vi "Page_Advanced_Initialize.vi"(6 "ctl references":T1, 8 "error in (no error)":errorcluster, 11 "AB_DLL in":refnum<class "AB_DLL.lvclass">) -> (0 "error out":errorcluster, 3 "AB_DLL out":refnum<class "AB_DLL.lvclass">)   [LabVIEW 2020, in "AB_DLL.lvclass"]
uses:
  <vilib>/AppBuilder/AB_Classes/DLL/AB_DLL.lvclass
  <resource>/Framework/Providers/Builds/AppBuilder/AB_UI_Page_Advanced_References.ctl
  <resource>/Framework/Providers/Common/provcom_StringGlobals.vi
  <vilib>/AppBuilder/AB_Classes/Application/AB_Application.lvclass
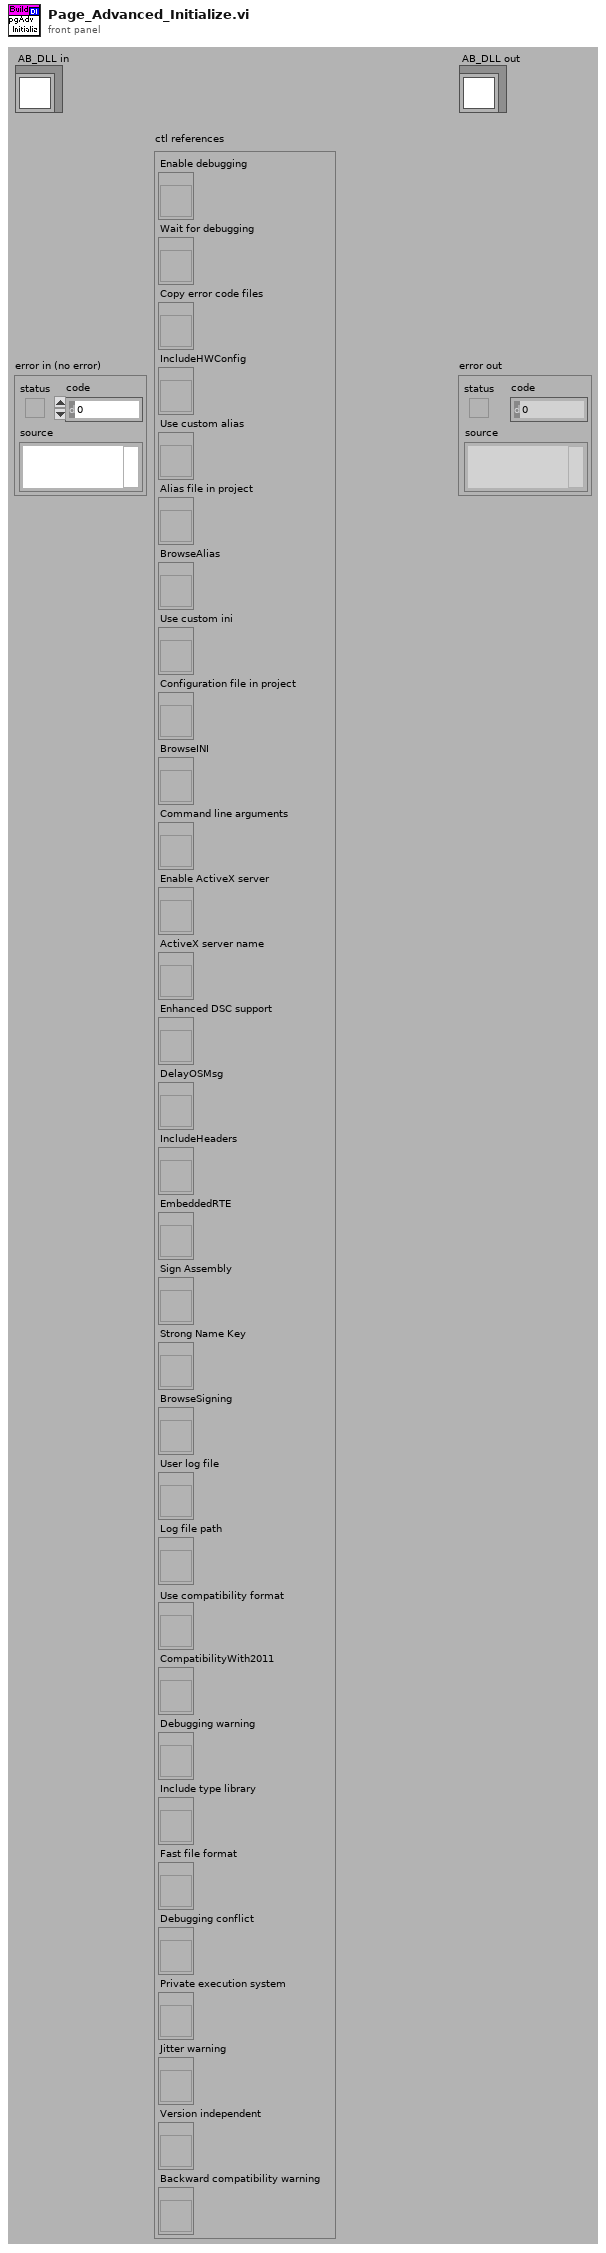
[diagram p1: front panel]
types:
  T1 = typedef "AB_UI_Page_Advanced_References.ctl" = cluster{"Enable debugging":refnum<vi>, "Wait for debugging":refnum<vi>, "Copy error code files":refnum<vi>, "IncludeHWConfig":refnum<vi>, "Use custom alias":refnum<vi>, "Alias file in project":refnum<vi>, "BrowseAlias":refnum<vi>, "Use custom ini":refnum<vi>, "Configuration file in project":refnum<vi>, "BrowseINI":refnum<vi>, "Command line arguments":refnum<vi>, "Enable ActiveX server":refnum<vi>, "ActiveX server name":refnum<vi>, "Enhanced DSC support":refnum<vi>, "DelayOSMsg":refnum<vi>, "IncludeHeaders":refnum<vi>, "EmbeddedRTE":refnum<vi>, "Sign Assembly":refnum<vi>, "Strong Name Key":refnum<vi>, "BrowseSigning":refnum<vi>, "User log file":refnum<vi>, "Log file path":refnum<vi>, "Use compatibility format":refnum<vi>, "CompatibilityWith2011":refnum<vi>, "Debugging warning":refnum<vi>, "Include type library":refnum<vi>, "Fast file format":refnum<vi>, "Debugging conflict":refnum<vi>, "Private execution system":refnum<vi>, "Jitter warning":refnum<vi>, "Version independent":refnum<vi>, "Backward compatibility warning":refnum<vi>}
  T2 = enum32{"invalid OS target", "Mac OS", "Windows 3.1", "Windows 95/NT", "Solaris 1", "Solaris 2", "HP-UX", "PowerMAX", "Linux", "Irix", "Rhapsody", "BeOS", "AIX", "OSF1", "VxWorks", "PharLap", "Carbon", "RTX", "Windows x64", "Linux x64", "Mac OS X x64"}
  T3 = typedef "LVRectTypeDef.ctl" = cluster{"Left":i16, "Top":i16, "Right":i16, "Bottom":i16}
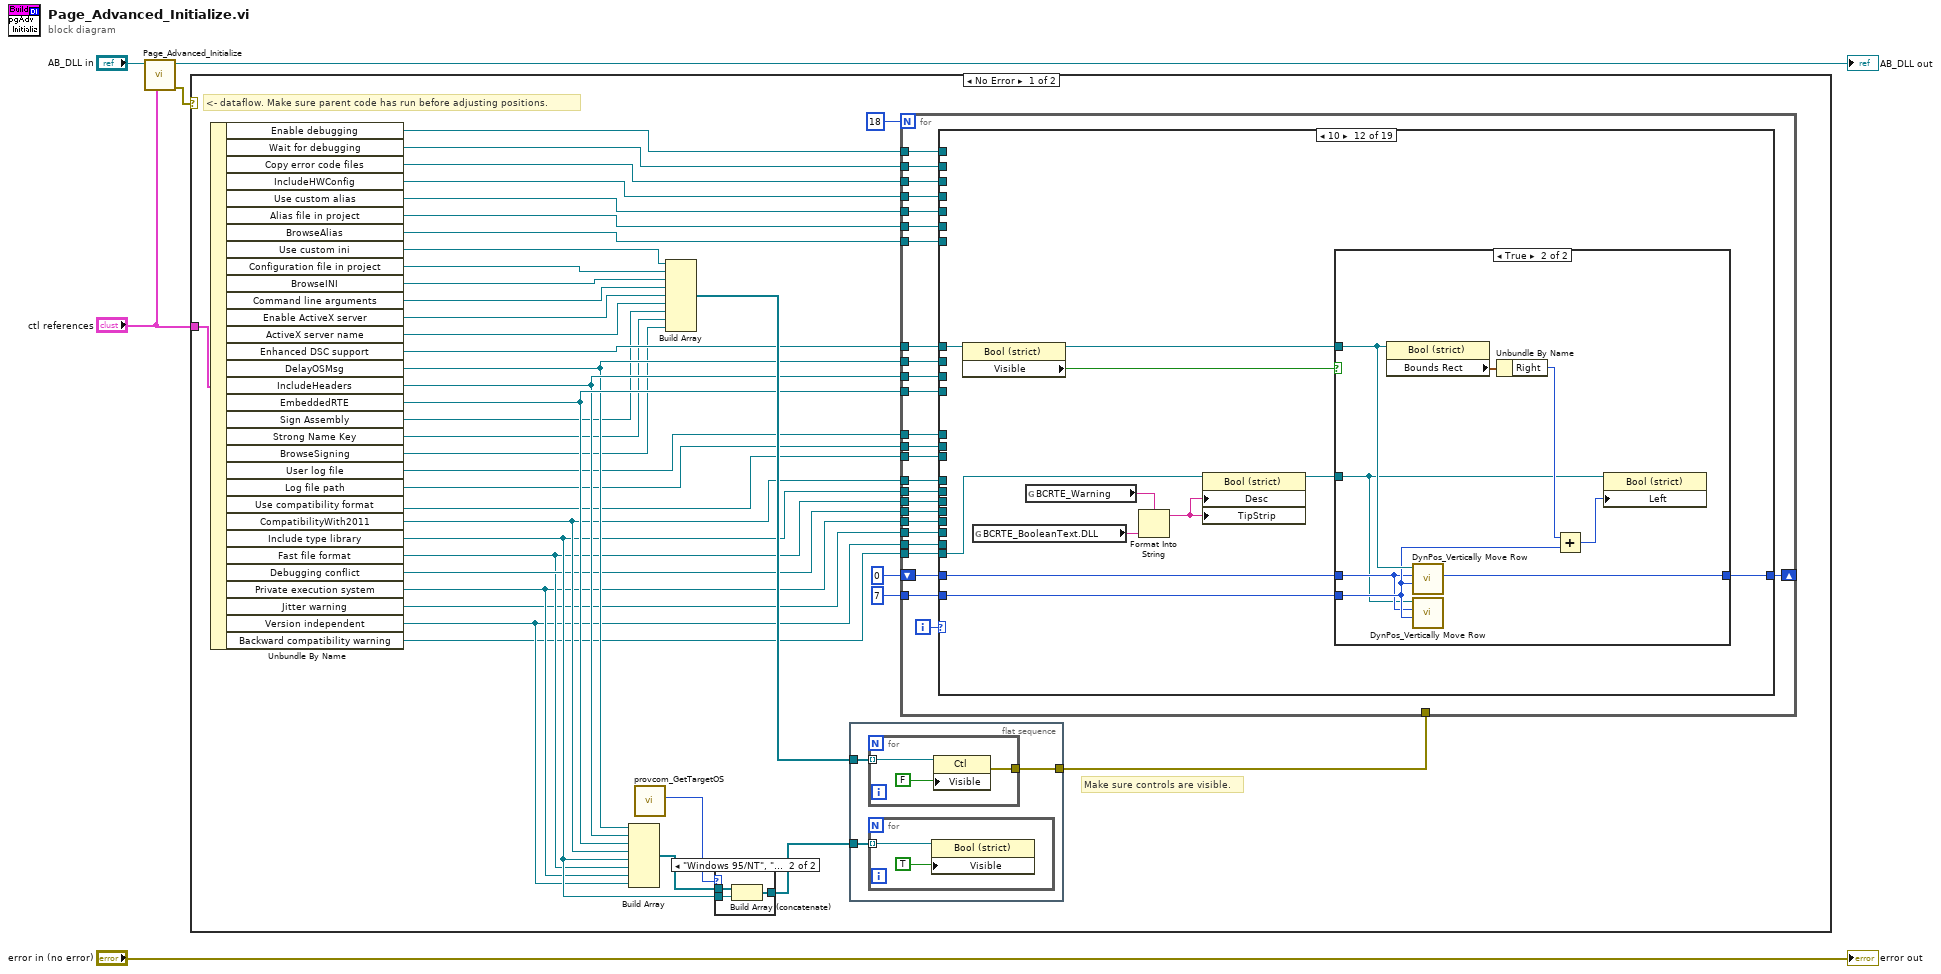
[diagram p0: block diagram]
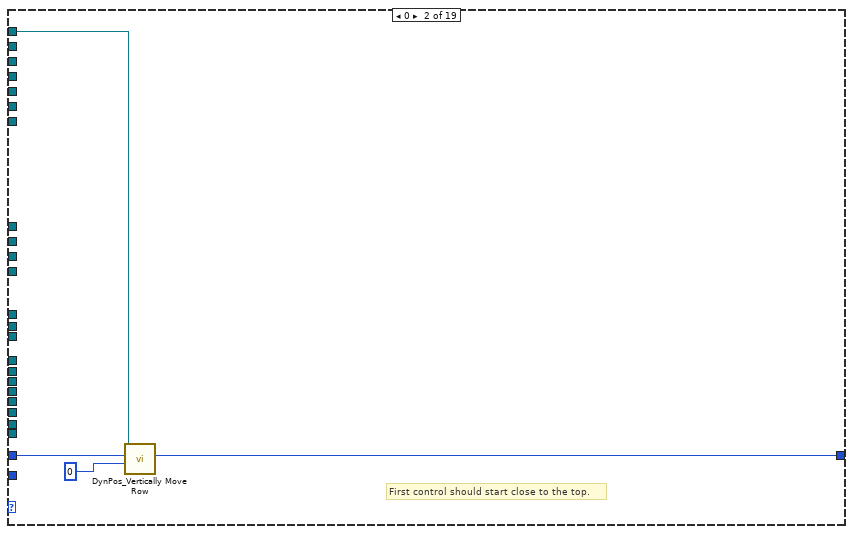
[diagram p4: hidden frame]
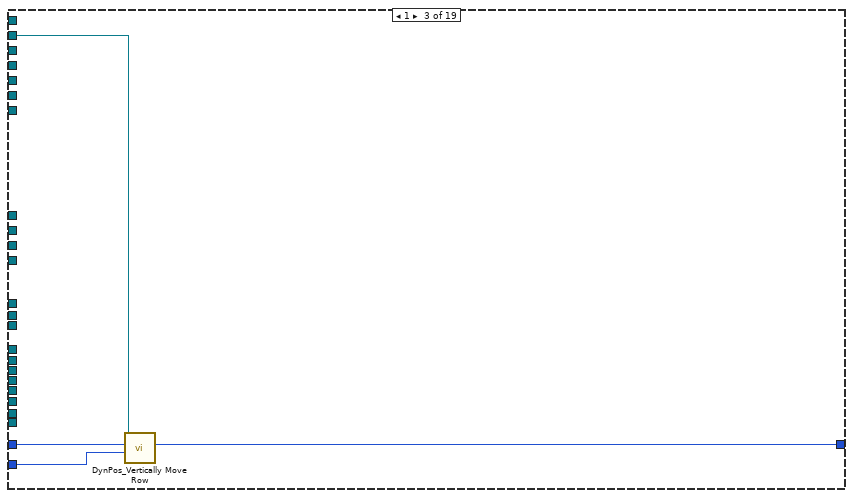
[diagram p5: hidden frame]
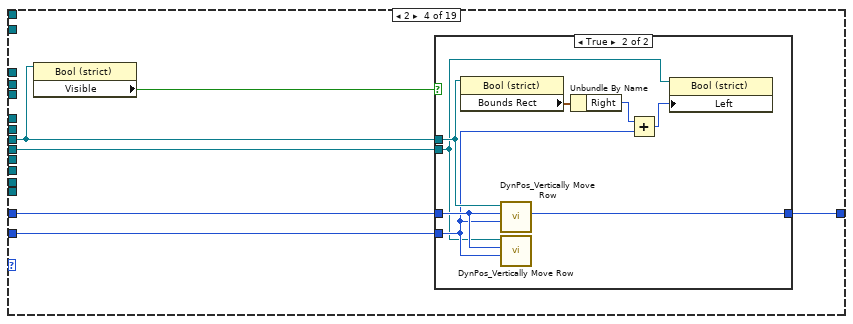
[diagram p6: hidden frame]
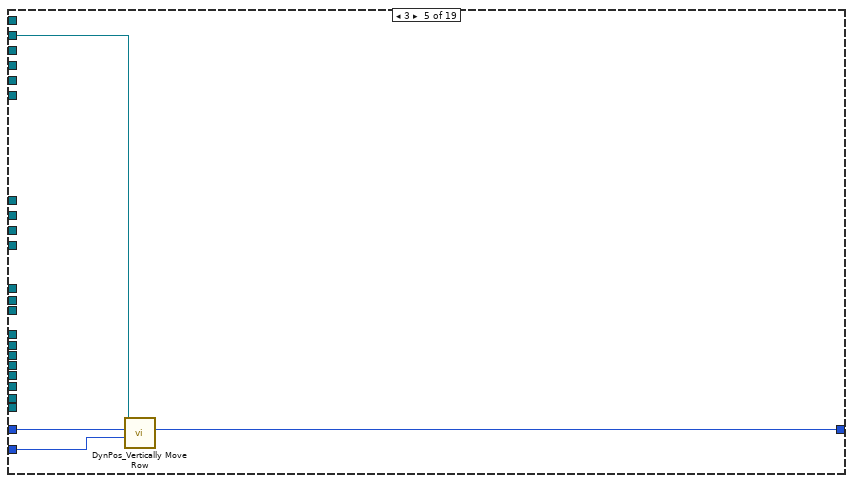
[diagram p8: hidden frame]
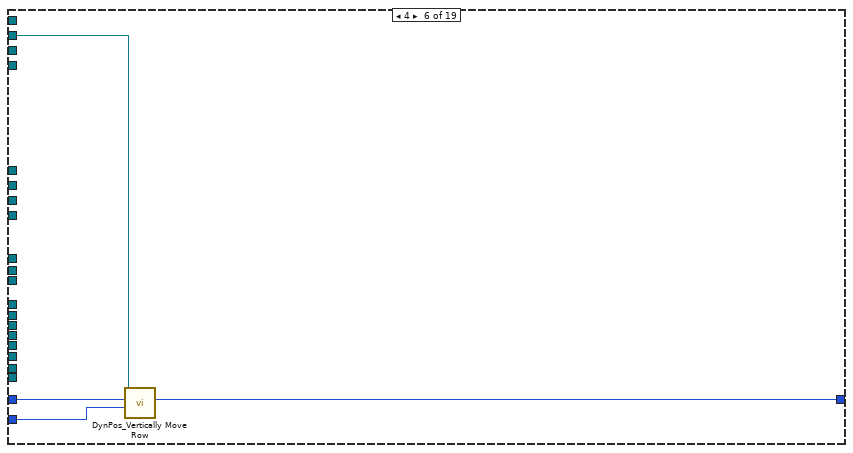
[diagram p9: hidden frame]
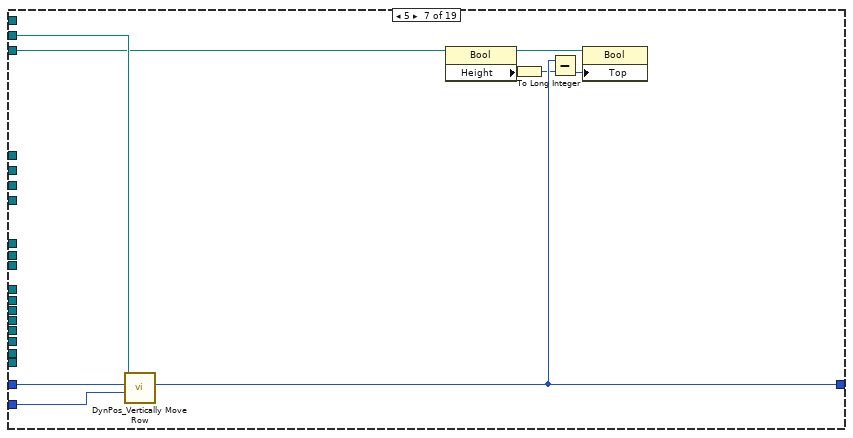
[diagram p10: hidden frame]
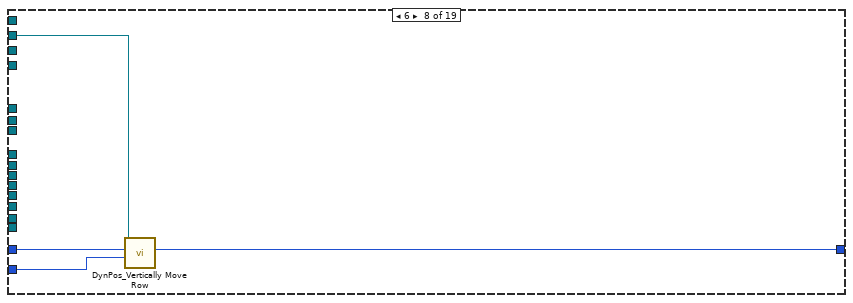
[diagram p11: hidden frame]
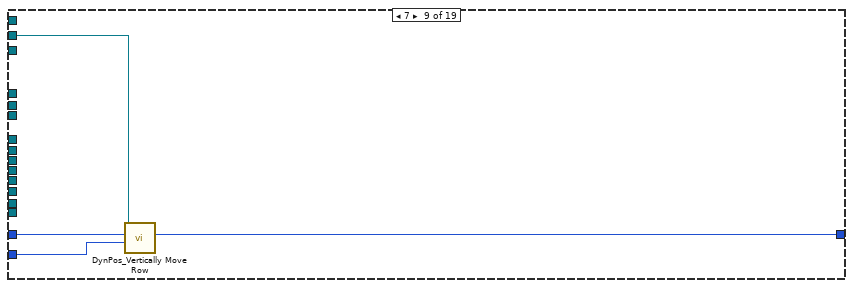
[diagram p12: hidden frame]
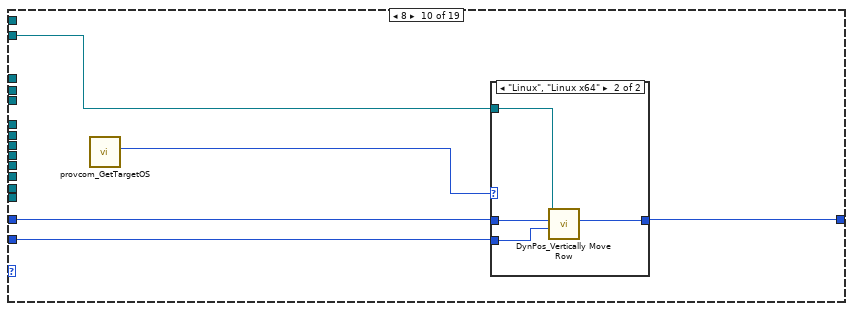
[diagram p13: hidden frame]
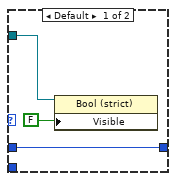
[diagram p14: hidden frame]
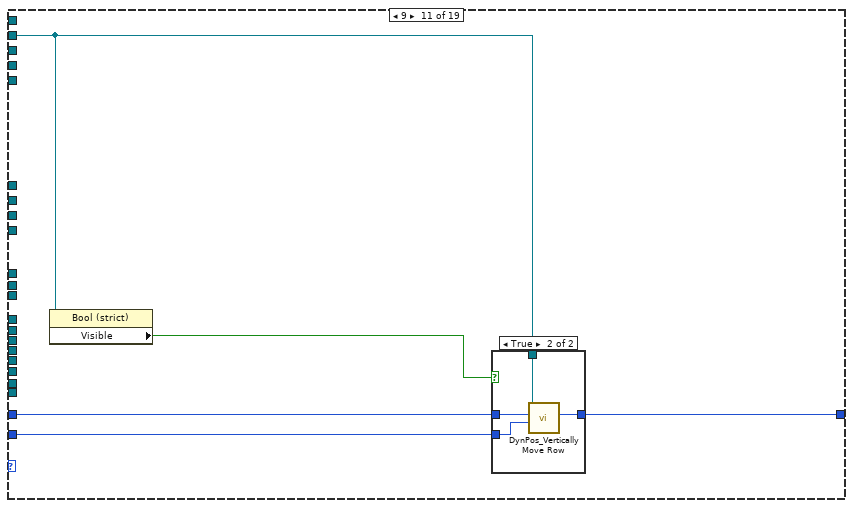
[diagram p15: hidden frame]
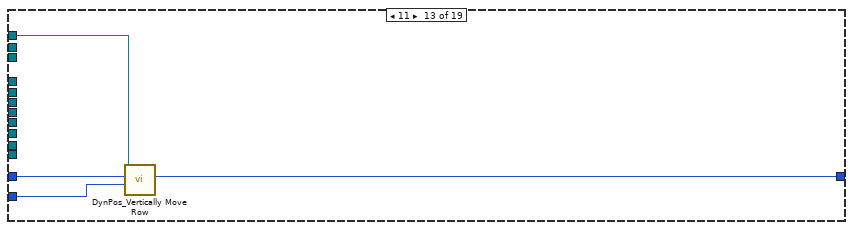
[diagram p18: hidden frame]
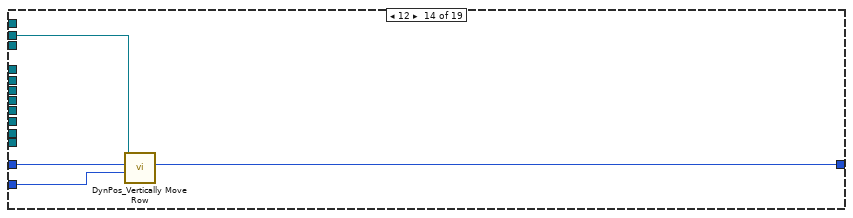
[diagram p19: hidden frame]
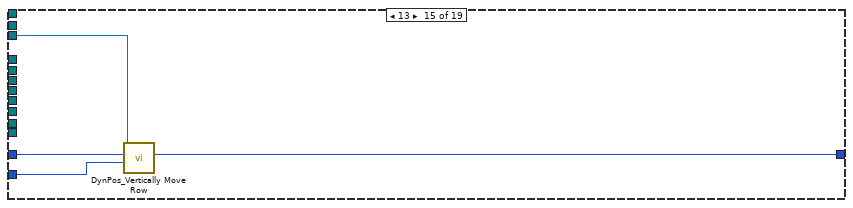
[diagram p20: hidden frame]
diagram:
  n1 = call-parent "Page_Advanced_Initialize.vi"("ctl references"="ctl references", "AB_Application in"="AB_DLL in") -> ("error out"=w1:errorcluster, "AB_Application out"=→"AB_DLL out":refnum<class "AB_DLL.lvclass">)  [unwired: 1 in, 7 out]
  n2 = case shown="No Error" w1 {
    tunnel: "ctl references" -> [w24 _]
    frame No Error {
      # "<- dataflow. Make sure parent code has run before adjusting positions."
      # "Make sure controls are visible."
      n3 = Unbundle By Name(w24) -> ("Enable debugging"=w45:refnum<vi>, "Wait for debugging"=w44:refnum<vi>, "Copy error code files"=w43:refnum<vi>, "IncludeHWConfig"=w42:refnum<vi>, "Use custom alias"=w41:refnum<vi>, "Alias file in project"=w40:refnum<vi>, "BrowseAlias"=w39:refnum<vi>, "Use custom ini"=w34:refnum<vi>, "Configuration file in project"=w33:refnum<vi>, "BrowseINI"=w32:refnum<vi>, "Command line arguments"=w31:refnum<vi>, "Enable ActiveX server"=w30:refnum<vi>, "ActiveX server name"=w29:refnum<vi>, "Enhanced DSC support"=w28:refnum<vi>, "DelayOSMsg"=w25:refnum<vi>, "IncludeHeaders"=w26:refnum<vi>, "EmbeddedRTE"=w27:refnum<vi>, "Sign Assembly"=w23:refnum<vi>, "Strong Name Key"=w22:refnum<vi>, "BrowseSigning"=w19:refnum<vi>, "User log file"=w21:refnum<vi>, "Log file path"=w20:refnum<vi>, "Use compatibility format"=w18:refnum<vi>, "CompatibilityWith2011"=w17:refnum<vi>, "Include type library"=w13:refnum<vi>, "Fast file format"=w10:refnum<vi>, "Debugging conflict"=w12:refnum<vi>, "Private execution system"=w9:refnum<vi>, "Jitter warning"=w8:refnum<vi>, "Version independent"=w7:refnum<vi>, "Backward compatibility warning"=w6:refnum<vi>)
      n4 = Build Array(w25, w26, w27, w17, w13, w10, w9, w7) -> (w16:refnum<vi>[])
      n5 = call <resource>:"provcom_GetTargetOS.vi"() -> ("App.TargetOS"=w14:T2)  [unwired: 11 in]
      n6 = Build Array(w34, w33, w32, w31, w30, w29, w23, w22, w19) -> (w35:refnum<vi>[])
      n7 = case shown="\"Windows 95/NT\", \"Windows x64\"" w14 {
        tunnel: w13 -> [_ w57]
        tunnel: w16 -> [w54 w56]
        tunnel: [w54 w55] -> w15
        frame Default {
        }
        frame "Windows 95/NT", "Windows x64" {
          n8 = Build Array (concatenate)(w56, w57) -> (w55:refnum<vi>[])
        }
      }
      n9 = flat-sequence {
        tunnel: w35 -> [w48]
        tunnel: w15 -> [w47]
        tunnel: [w46] -> w11
        frame #0 {
          n10 = for {
            tunnel: w48 -> [w53] mode=indexing
            tunnel: [w51] -> w46
            n11 = property class="Ctl"(reference=w53, "Visible"=FALSE) -> (error out=w51:errorcluster)  [unwired: 1 in, 1 out]
          }
          n12 = for {
            tunnel: w47 -> [w50] mode=indexing
            n13 = property class="Bool (strict)"(reference=w50, "Visible"=TRUE) -> ()  [unwired: 1 in, 2 out]
          }
        }
      }
      n14 = for {
        N: 18 -> [_]
        tunnel: w45 -> [w82]
        tunnel: w44 -> [w81]
        tunnel: w43 -> [w80]
        tunnel: w42 -> [w79]
        tunnel: w41 -> [w78]
        tunnel: w40 -> [w77]
        tunnel: w39 -> [w76]
        shift-right: [w73] -> _
        shift-left: 0 ("Bottom of last control") -> [w75]
        tunnel: 7 ("Bottom of last control") -> [w74]
        tunnel: w25 -> [w72]
        tunnel: w26 -> [w71]
        tunnel: w27 -> [w70]
        tunnel: w28 -> [w69]
        tunnel: w21 -> [w68]
        tunnel: w20 -> [w67]
        tunnel: w18 -> [w66]
        tunnel: w17 -> [w65]
        tunnel: w13 -> [w64]
        tunnel: w10 -> [w63]
        tunnel: w12 -> [w62]
        tunnel: w11 -> [_]
        tunnel: w9 -> [w61]
        tunnel: w8 -> [w60]
        tunnel: w7 -> [w59]
        tunnel: w6 -> [w58]
        i -> [w83]
        n15 = case shown="10" w83 {
          tunnel: w82 -> [_ w87 _ _ _ _ _ _ _ _ _ _ _ _ _ _ _ _ _]
          tunnel: w81 -> [_ _ w89 _ _ _ _ _ _ _ _ _ _ _ _ _ _ _ _]
          tunnel: w80 -> [_ _ _ _ w108 _ _ _ _ _ _ _ _ _ _ _ _ _ _]
          tunnel: w79 -> [_ _ _ _ _ _ _ _ _ _ w145 _ _ _ _ _ _ _ _]
          tunnel: w78 -> [_ _ _ _ _ w112 _ _ _ _ _ _ _ _ _ _ _ _ _]
          tunnel: w77 -> [_ _ _ _ _ _ w122 _ _ _ _ _ _ _ _ _ _ _ _]
          tunnel: w76 -> [_ _ _ _ _ _ w121 _ _ _ _ _ _ _ _ _ _ _ _]
          tunnel: w75 -> [w84 w88 w92 w97 w111 w115 w124 w128 w132 w137 w148 w164 w178 w182 w186 w189 w194 w202 w208]
          tunnel: w74 -> [_ _ w91 w96 w110 w114 w123 w127 w131 w136 w147 w163 w177 w181 w185 w188 w193 w201 w207]
          tunnel: [w84 w86 w90 w98 w109 w113 w117 w126 w130 w135 w146 w162 w176 w180 w184 w187 w192 w200 w206] -> w73
          tunnel: w72 -> [_ _ _ _ _ _ _ w125 _ _ _ _ _ _ _ _ _ _ _]
          tunnel: w71 -> [_ _ _ _ _ _ _ _ w129 _ _ _ _ _ _ _ _ _ _]
          tunnel: w70 -> [_ _ _ _ _ _ _ _ _ w134 _ _ _ _ _ _ _ _ _]
          tunnel: w69 -> [_ _ _ _ _ _ _ _ _ _ _ w161 _ _ _ _ _ _ _]
          tunnel: w68 -> [_ _ _ _ _ _ _ _ _ _ _ _ w175 _ _ _ _ _ _]
          tunnel: w67 -> [_ _ _ _ _ _ _ _ _ _ _ _ _ w179 _ _ _ _ _]
          tunnel: w66 -> [_ _ _ _ _ _ _ _ _ _ _ _ _ _ w183 _ _ _ _]
          tunnel: w65 -> [_ _ _ _ _ _ _ _ _ _ _ _ _ _ _ w190 _ _ _]
          tunnel: w64 -> [_ _ _ _ _ _ _ _ _ _ _ _ _ _ _ _ w191 _ _]
          tunnel: w63 -> [_ _ _ w93 _ _ _ _ _ _ _ _ _ _ _ _ _ _ _]
          tunnel: w62 -> [_ _ _ w95 _ _ _ _ _ _ _ _ _ _ _ _ _ _ _]
          tunnel: w61 -> [_ _ _ _ _ _ _ _ _ _ _ _ _ _ _ _ _ w199 _]
          tunnel: w60 -> [_ _ _ _ _ _ _ _ _ _ _ _ _ _ _ _ _ w198 _]
          tunnel: w59 -> [_ _ _ _ _ _ _ _ _ _ _ _ _ _ _ _ _ _ w209]
          tunnel: w58 -> [_ _ _ _ _ _ _ _ _ _ _ w156 _ _ _ _ _ _ _]
          frame Default {
          }
          frame 0 {
            # "First control should start close to the top."
            n16 = call <vilib>:"DynPos_Vertically Move Row.vi"("Pixel separation (6)"=0, "Bottom of last control"=w88, "Control"=w87) -> ("Bottom pixel"=w86:i32)  [unwired: 1 in, 7 out]
          }
          frame 1 {
            n17 = call <vilib>:"DynPos_Vertically Move Row.vi"("Pixel separation (6)"=w91, "Bottom of last control"=w92, "Control"=w89) -> ("Bottom pixel"=w90:i32)  [unwired: 1 in, 7 out]
          }
          frame 2 {
            n18 = property class="Bool (strict)"(reference=w93) -> ("Visible"=w94:bool)  [unwired: 1 in, 2 out]
            n19 = case shown="True" w94 {
              tunnel: [w99 w107] -> w98
              tunnel: w97 -> [w99 w106]
              tunnel: w93 -> [_ w105]
              tunnel: w96 -> [_ w102]
              tunnel: w95 -> [_ w101]
              frame False {
              }
              frame True {
                n20 = property class="Bool (strict)"(reference=w105) -> ("Bounds Rect"=w104:T3)  [unwired: 1 in, 2 out]
                n21 = call <vilib>:"DynPos_Vertically Move Row.vi"("Pixel separation (6)"=w102, "Bottom of last control"=w106, "Control"=w105) -> ("Bottom pixel"=w107:i32)  [unwired: 1 in, 7 out]
                n22 = call <vilib>:"DynPos_Vertically Move Row.vi"("Pixel separation (6)"=w102, "Bottom of last control"=w106, "Control"=w101) -> ()  [unwired: 1 in, 8 out]
                n23 = Unbundle By Name(w104) -> ("Right"=w103:i16)
                n24 = Add(x=w103, y=w102) -> (x+y=w100:i32)
                n25 = property class="Bool (strict)"(reference=w101, "Left"=w100) -> ()  [unwired: 1 in, 2 out]
              }
            }
          }
          frame 3 {
            n26 = call <vilib>:"DynPos_Vertically Move Row.vi"("Pixel separation (6)"=w110, "Bottom of last control"=w111, "Control"=w108) -> ("Bottom pixel"=w109:i32)  [unwired: 1 in, 7 out]
          }
          frame 4 {
            n27 = call <vilib>:"DynPos_Vertically Move Row.vi"("Pixel separation (6)"=w114, "Bottom of last control"=w115, "Control"=w112) -> ("Bottom pixel"=w113:i32)  [unwired: 1 in, 7 out]
          }
          frame 5 {
            n28 = call <vilib>:"DynPos_Vertically Move Row.vi"("Pixel separation (6)"=w123, "Bottom of last control"=w124, "Control"=w122) -> ("Bottom pixel"=w117:i32)  [unwired: 1 in, 7 out]
            n29 = property class="Bool"(reference=w121) -> (reference out=w120:refnum<vi>, "Height"=w119:u32)  [unwired: 1 in, 1 out]
            n30 = To Long Integer(number=w119) -> (32bit integer=w116:i32)
            n31 = Subtract(x=w117, y=w116) -> (x-y=w118:i32)
            n32 = property class="Bool"(reference=w120, "Top"=w118) -> ()  [unwired: 1 in, 2 out]
          }
          frame 6 {
            n33 = call <vilib>:"DynPos_Vertically Move Row.vi"("Pixel separation (6)"=w127, "Bottom of last control"=w128, "Control"=w125) -> ("Bottom pixel"=w126:i32)  [unwired: 1 in, 7 out]
          }
          frame 7 {
            n34 = call <vilib>:"DynPos_Vertically Move Row.vi"("Pixel separation (6)"=w131, "Bottom of last control"=w132, "Control"=w129) -> ("Bottom pixel"=w130:i32)  [unwired: 1 in, 7 out]
          }
          frame 8 {
            n35 = call <resource>:"provcom_GetTargetOS.vi"() -> ("App.TargetOS"=w133:T2)  [unwired: 11 out]
            n36 = case shown="\"Linux\", \"Linux x64\"" w133 {
              tunnel: w137 -> [w140 w144]
              tunnel: w136 -> [_ w143]
              tunnel: [w140 w142] -> w135
              tunnel: w134 -> [w139 w141]
              frame Default {
                n37 = property class="Bool (strict)"(reference=w139, "Visible"=FALSE) -> ()  [unwired: 1 in, 2 out]
              }
              frame "Linux", "Linux x64" {
                n38 = call <vilib>:"DynPos_Vertically Move Row.vi"("Pixel separation (6)"=w143, "Bottom of last control"=w144, "Control"=w141) -> ("Bottom pixel"=w142:i32)  [unwired: 1 in, 7 out]
              }
            }
          }
          frame 9 {
            n39 = property class="Bool (strict)"(reference=w145) -> ("Visible"=w149:bool)  [unwired: 1 in, 2 out]
            n40 = case shown="True" w149 {
              tunnel: w148 -> [w150 w154]
              tunnel: w147 -> [_ w153]
              tunnel: [w150 w152] -> w146
              tunnel: w145 -> [_ w151]
              frame False {
              }
              frame True {
                n41 = call <vilib>:"DynPos_Vertically Move Row.vi"("Pixel separation (6)"=w153, "Bottom of last control"=w154, "Control"=w151) -> ("Bottom pixel"=w152:i32)  [unwired: 1 in, 7 out]
              }
            }
          }
          frame 10 {
            n42 = property class="Bool (strict)"(reference=w161) -> (reference out=w160:refnum<vi>, "Visible"=w165:bool)  [unwired: 1 in, 1 out]
            n43 = global read "provcom_StringGlobals.vi" "BCRTE_BooleanText.DLL"() -> (w158:string)
            n44 = global read "provcom_StringGlobals.vi" "BCRTE_Warning"() -> (w157:string)
            n45 = Format Into String(format string=w157, w158) -> (resulting string=w159:string)  [unwired: 2 in, 1 out]
            n46 = property class="Bool (strict)"(reference=w156, "Desc"=w159, "TipStrip"=w159) -> (reference out=w155:refnum<vi>)  [unwired: 1 in, 1 out]
            n47 = case shown="True" w165 {
              tunnel: w164 -> [w166 w168]
              tunnel: w163 -> [_ w169]
              tunnel: [w166 w171] -> w162
              tunnel: w160 -> [_ w170]
              tunnel: w155 -> [_ w167]
              frame False {
              }
              frame True {
                n48 = property class="Bool (strict)"(reference=w170) -> ("Bounds Rect"=w174:T3)  [unwired: 1 in, 2 out]
                n49 = call <vilib>:"DynPos_Vertically Move Row.vi"("Pixel separation (6)"=w169, "Bottom of last control"=w168, "Control"=w170) -> ("Bottom pixel"=w171:i32)  [unwired: 1 in, 7 out]
                n50 = call <vilib>:"DynPos_Vertically Move Row.vi"("Pixel separation (6)"=w169, "Bottom of last control"=w168, "Control"=w167) -> ()  [unwired: 1 in, 8 out]
                n51 = Unbundle By Name(w174) -> ("Right"=w173:i16)
                n52 = Add(x=w173, y=w169) -> (x+y=w172:i32)
                n53 = property class="Bool (strict)"(reference=w167, "Left"=w172) -> ()  [unwired: 1 in, 2 out]
              }
            }
          }
          frame 11 {
            n54 = call <vilib>:"DynPos_Vertically Move Row.vi"("Pixel separation (6)"=w177, "Bottom of last control"=w178, "Control"=w175) -> ("Bottom pixel"=w176:i32)  [unwired: 1 in, 7 out]
          }
          frame 12 {
            n55 = call <vilib>:"DynPos_Vertically Move Row.vi"("Pixel separation (6)"=w181, "Bottom of last control"=w182, "Control"=w179) -> ("Bottom pixel"=w180:i32)  [unwired: 1 in, 7 out]
          }
          frame 13 {
            n56 = call <vilib>:"DynPos_Vertically Move Row.vi"("Pixel separation (6)"=w185, "Bottom of last control"=w186, "Control"=w183) -> ("Bottom pixel"=w184:i32)  [unwired: 1 in, 7 out]
          }
          frame 14 {
            n57 = call <vilib>:"DynPos_Vertically Move Row.vi"("Pixel separation (6)"=w188, "Bottom of last control"=w189, "Control"=w190) -> ("Bottom pixel"=w187:i32)  [unwired: 1 in, 7 out]
          }
          frame 15 {
            n58 = call <vilib>:"DynPos_Vertically Move Row.vi"("Pixel separation (6)"=w193, "Bottom of last control"=w194, "Control"=w191) -> ("Bottom pixel"=w192:i32)  [unwired: 1 in, 7 out]
          }
          frame 16 {
            n59 = property class="Bool (strict)"(reference=w199) -> ("Bounds Rect"=w197:T3)  [unwired: 1 in, 2 out]
            n60 = call <vilib>:"DynPos_Vertically Move Row.vi"("Pixel separation (6)"=w201, "Bottom of last control"=w202, "Control"=w199) -> ("Bottom pixel"=w200:i32)  [unwired: 1 in, 7 out]
            n61 = call <vilib>:"DynPos_Vertically Move Row.vi"("Pixel separation (6)"=w201, "Bottom of last control"=w202, "Control"=w198) -> ()  [unwired: 1 in, 8 out]
            n62 = Unbundle By Name(w197) -> ("Right"=w196:i16)
            n63 = Add(x=w196, y=w201) -> (x+y=w195:i32)
            n64 = property class="Bool (strict)"(reference=w198, "Left"=w195) -> ()  [unwired: 1 in, 2 out]
          }
          frame 17 {
            n65 = global read "provcom_StringGlobals.vi" "BCRTE_BooleanText.DLL"() -> (w204:string)
            n66 = global read "provcom_StringGlobals.vi" "BCRTE_Description.DLL"() -> (w203:string)
            n67 = property class="Bool (strict)"(reference=w209, "BoolText.Text"=w204, "Desc"=w203) -> (reference out=w205:refnum<vi>, "Visible"=w210:bool)  [unwired: 1 in, 1 out]
            n68 = case shown="True" w210 {
              tunnel: w208 -> [w211 w215]
              tunnel: w207 -> [_ w214]
              tunnel: [w211 w213] -> w206
              tunnel: w205 -> [_ w212]
              frame False {
              }
              frame True {
                n69 = call <vilib>:"DynPos_Vertically Move Row.vi"("Pixel separation (6)"=w214, "Bottom of last control"=w215, "Control"=w212) -> ("Bottom pixel"=w213:i32)  [unwired: 1 in, 7 out]
              }
            }
          }
        }
      }
    }
    frame Error {
    }
  }
  "error out" <- "error in (no error)"
